vi "PPMSDR_Parent_single.vi"() -> ()   [LabVIEW 2016]
uses:
  <vilib>/lvdsc/historical/Open Trace (Numeric).vi
  <vilib>/lvdsc/historical/Write Trace (Numeric).vi
  <vilib>/lvdsc/NI_DSC.lvlib
panel:
  in  "pattern":string="logppmsdata*"
  in  "Folder Path In":path=path "C:/Users/Pittsburgh/Desktop/DRLOG"
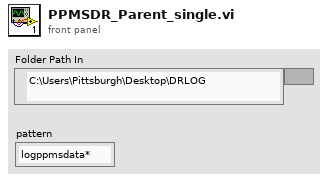
[diagram p1: front panel]
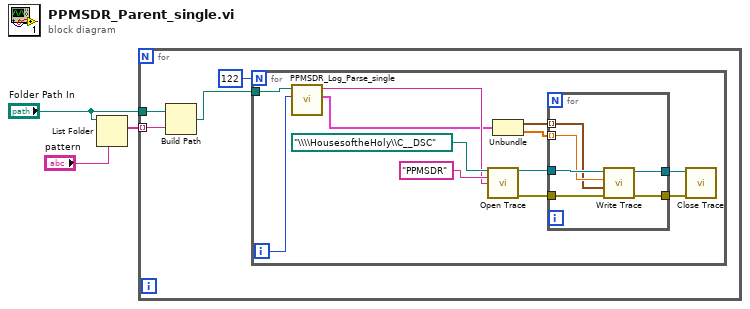
[diagram p0: block diagram]
diagram:
  n1 = List Folder(path="Folder Path In", pattern="pattern") -> (filenames=w2:string[])  [unwired: 2 in, 3 out]
  n2 = for {
    tunnel: w2 -> [w7] mode=indexing
    tunnel: "Folder Path In" -> [w6]
    n3 = Build Path(base path=w6, name or relative path=w7) -> (appended path=w5:path)
    n4 = for {
      N: 122 -> [_]
      tunnel: w5 -> [w8]
      i -> [w11]
      n5 = call "PPMSDR_Log_Parse_single.vi"("index"=w11, "file path (dialog if empty)"=w8) -> ("XY Graph"=w9:cluster{timestamp[], dbl[]}, "element"=w10:string)  [unwired: 8 in]
      n6 = call-poly <vilib>:"Open Trace.vi"("database URL"=path "\\\\HousesoftheHoly\\C__DSC", "process name"="PPMSDR", "trace name"=w10) -> ("trace reference"=w15:refnum<k1>, "error out"=w14:errorcluster)  [unwired: 10 in, 1 out]
      n7 = Unbundle(w9) -> (w13:timestamp[], w12:dbl[])
      n8 = for {
        tunnel: [w25] -> w17
        tunnel: [w24] -> w16
        tunnel: w15 -> [w23]
        tunnel: w14 -> [w22]
        tunnel: w13 -> [w20] mode=indexing
        tunnel: w12 -> [w21] mode=indexing
        n9 = call-poly <vilib>:"Write Trace.vi"("error in (no error)"=w22, "timestamp (now)"=w20, "value"=w21, "trace ref"=w23) -> ("error out"=w25:errorcluster, "trace ref out"=w24:refnum<k1>)  [unwired: 6 in]
      }
      n10 = call <vilib>:"Close Trace.vi"("error in (no error)"=w17, "trace reference"=w16) -> ()  [unwired: 9 in, 1 out]
    }
  }
